vi "Emballage_BDD_choix_Config.vi"(8 "Error in":errorcluster caption="Error in (no error)") -> (0 "Error out":errorcluster, 1 "Arrêt programme?":bool=TRUE, 2 "Produit code FAS OUT":string, 3 "CLS_param_produit":T1)   [LabVIEW 2020]
uses:
  Emballage_BDD_param_Produit.ctl
  Choix_Config_ref.ctl
  Modules/FS/60_FS_Controles/60_FS_SetGet.ctl
  Labview emballage/enum_ON_OFF_Lecteur.ctl
  <vilib>/Utility/miscctls.llb/LVRowAndColumnUnsignedTypeDef.ctl
  <vilib>/drjdpowell/SQLite Library/SQL Connection/Open (path).vi
  <vilib>/drjdpowell/SQLite Library/SQL Connection/Open (string).vi
  <vilib>/AdvancedString/Path To Command Line String.vi
  <vilib>/drjdpowell/SQLite Library/SQL Connection/Connection.lvclass
panel:
  out "Indice Imprimante":i32
  in  "Port Com scan":u16(ring) items=["Autre", "FLATPROP"]
  out "imprimante Etiquettes":string(combo)="Sans_imprimante"
  out "Glissière":u8(slide) scale=0.0..100.0
  out "Dernière Synchro.":timestamp
  out "OK":bool
  in  "Bouton synchroniser":bool
  in  "Bouton Imprimante":bool
  in  "Bouton scanner":bool
  out "Produit code FAS":string
  out "sous-tableau":string[](array[string])
  in  "Bouton OK":bool
  in  "where valeur":string[](array[string])
  in  "Where colonne":string[](array[string])
  in  "stop":bool
  in  "Famille":u16(ring) items=["", "CHIPREG", "F011106", "F011107", "FASPROP", "FLATPROP", "NoTest", "S0020002", "S0020010", "S1121065", "S1121066", "S1121229", "S1121289", "S1121437", "S1210017", "S1220009", "S1220096"]
  in  "designation":u16(ring) items=["", "104mA_230Ohm", "138mA_130Ohm", "167mA 72ohm", "16mA_1152Ohm", "182mA_57Ohm", "186mA_14.4Ohm", "18V DC   4.50W", "18mA 288ohm", "211mA_57Ohm", "21mA 1152ohm", "21mA_1152Ohm", "23mA_576Ohm", "24V DC 4/0.40W", "258 SDGNUL  24V DC  14.50W", "264mA_36Ohm", "29mA 576ohm", "32mA 288ohm", "354mA_20Ohm", "36mA_230Ohm", "417mA_14.4Ohm", "4212 SDGNUL  24V DC  10W", "42mA 288ohm", "42mA_288Ohm", "48mA_130Ohm", "500mA_10Ohm", "59mA_288Ohm", "62mA_130Ohm", "83mA 72ohm", "83mA_72Ohm", "88mA_130Ohm", "BLOC  1P CHIPREG 10 l/min G1/8'' ", "BLOC  1P CHIPREG 10 l/min G1/8'' CLEAN ", "BLOC  1P CHIPREG 10 l/min M.MOUNT ", "BLOC  1P CHIPREG 10 l/min M.MOUNT CLEAN ", "BLOC  1P CHIPREG 500 ml/min G1/8 ", "BLOC  1P CHIPREG 500 ml/min G1/8 CLEAN ", "BLOC  1P CHIPREG 500 ml/min M.MOUNT ", "BLOC  1P CHIPREG 500 ml/min M.MOUNT CLEAN ", "BLOC  4P TAEMA EXTEND  24V / 5V DC", "BLOC 11-211P604-H0 4P 2 NIPPEL INJ ", "BLOC 2P TRILOGY ACTIVE EXHALATION CONTROL MODULE ", "BLOC 2X8P 3/2 NC NIPPEL ALU ", "BLOC 3P CALIBRATION UNIT ", "BLOC 4P EVU SN ELITE P4C HYBRID ", "BLOC 4P MANIFOLD VENTILATOR ", "BLOC 5P ARGON-N2 GASBOX FOR PQMS ", "BLOC 8P 3/2 NC NIPPEL ALU ", "BLOC DAGMAR DIGITAL ", "CARINA  AVEC FILTRE FERRITE ET GOUPILLE ", "CHIPREG MFC, 1 ls/min, RS232, G1/8, AIR, A-CLEAN ", "CHIPREG MFC, 1 ls/min, RS232, G1/8, AIR, STD MEDIC ", "CHIPREG MFC, 1 ls/min, RS232, M.MOUNT, AIR, A-CLEAN ", "CHIPREG MFC, 1 ls/min, RS232, M.MOUNT, AIR,STD MEDIC ", "CHIPREG MFC, 1 ls/min, RS485, G1/8, AIR, A-CLEAN ", "CHIPREG MFC, 1 ls/min, RS485, G1/8, AIR, STD MEDIC ", "CHIPREG MFC, 1 ls/min, RS485, M.MOUNT, AIR, A-CLEAN ", "CHIPREG MFC, 1 ls/min, RS485, M.MOUNT, AIR,STD MEDIC ", "CHIPREG MFC, 10 ls/min, RS232, G1/8, AIR, A-CLEAN ", "CHIPREG MFC, 10 ls/min, RS232, G1/8, AIR, STD MEDIC ", "CHIPREG MFC, 10 ls/min, RS232, M.MOUNT, AIR, A-CLEAN ", "CHIPREG MFC, 10 ls/min, RS232, M.MOUNT, AIR, STD MEDIC ", "CHIPREG MFC, 10 ls/min, RS485, G1/8, AIR, A-CLEAN ", "CHIPREG MFC, 10 ls/min, RS485, G1/8, AIR, STD MEDIC ", "CHIPREG MFC, 10 ls/min, RS485, M.MOUNT, AIR, A-CLEAN ", "CHIPREG MFC, 10 ls/min, RS485, M.MOUNT, AIR, STD MEDIC ", "CHIPREG MFC, 2 ls/min, RS232, G1/8, AIR, A-CLEAN ", "CHIPREG MFC, 2 ls/min, RS232, G1/8, AIR, STD MEDIC ", "CHIPREG MFC, 2 ls/min, RS232, M.MOUNT, AIR, A-CLEAN ", "CHIPREG MFC, 2 ls/min, RS232, M.MOUNT, AIR,STD MEDIC ", "CHIPREG MFC, 2 ls/min, RS485, G1/8, AIR, A-CLEAN ", "CHIPREG MFC, 2 ls/min, RS485, G1/8, AIR, STD MEDIC ", "CHIPREG MFC, 2 ls/min, RS485, M.MOUNT, AIR, A-CLEAN ", "CHIPREG MFC, 2 ls/min, RS485, M.MOUNT, AIR,STD MEDIC ", "CHIPREG MFC, 200 mls/min, RS232, G1/8, AIR, A-CLEAN ", "CHIPREG MFC, 200 mls/min, RS232, G1/8, AIR, STD MEDIC ", "CHIPREG MFC, 200 mls/min, RS232, M.MOUNT, AIR, A-CLEAN ", "CHIPREG MFC, 200 mls/min, RS232, M.MOUNT, AIR,STD MEDIC ", "CHIPREG MFC, 200 mls/min, RS485, G1/8, AIR, A-CLEAN ", "CHIPREG MFC, 200 mls/min, RS485, G1/8, AIR, STD MEDIC ", "CHIPREG MFC, 200 mls/min, RS485, M.MOUNT, AIR, A-CLEAN ", "CHIPREG MFC, 200 mls/min, RS485, M.MOUNT, AIR,STD MEDIC ", "CHIPREG MFC, 5 ls/min, RS232, G1/8, AIR, A-CLEAN ", "CHIPREG MFC, 5 ls/min, RS232, G1/8, AIR, STD MEDIC ", "CHIPREG MFC, 5 ls/min, RS232, M.MOUNT, AIR, A-CLEAN ", "CHIPREG MFC, 5 ls/min, RS232, M.MOUNT, AIR,STD MEDIC ", "CHIPREG MFC, 5 ls/min, RS485, G1/8, AIR, A-CLEAN ", "CHIPREG MFC, 5 ls/min, RS485, G1/8, AIR, STD MEDIC ", "CHIPREG MFC, 5 ls/min, RS485, M.MOUNT, AIR, A-CLEAN ", "CHIPREG MFC, 5 ls/min, RS485, M.MOUNT, AIR,STD MEDIC ", "CHIPREG MFC, 500 mls/min, RS232, G1/8, AIR, A-CLEAN ", "CHIPREG MFC, 500 mls/min, RS232, G1/8, AIR, STD MEDIC ", "CHIPREG MFC, 500 mls/min, RS232, M.MOUNT, AIR, A-CLEAN ", "CHIPREG MFC, 500 mls/min, RS232, M.MOUNT, AIR,STD MEDIC ", "CHIPREG MFC, 500 mls/min, RS485, G1/8, AIR, A-CLEAN ", "CHIPREG MFC, 500 mls/min, RS485, G1/8, AIR, STD MEDIC ", "CHIPREG MFC, 500 mls/min, RS485, M.MOUNT, AIR, A-CLEAN ", "CHIPREG MFC, 500 mls/min, RS485, M.MOUNT, AIR,STD MEDIC ", "DOSIERPATRONE (AUSTAUSCH-SET) ", "ENSEMBLE TORON EV PURGE & PEP ", "ENSEMBLE TORON EVS PEP N° KY724000 ", "ENSEMBLE TORON EVS PEP N° ST080387 D ", "Fluid control Current controller 211mA 24V IN4-20mA/IN10V ", "M06    18V DC   4.50W", "M06  5/1.5V DC 4.2/0.4W", "MODULE 1P CURRENT CTRL, SETPOINT 4-20mA ", "REVOLVER X6 "]
  in  "suffixe":u16(ring) items=["", "       ", "1110000", "1210000", "A      ", "D2MFIL", "D2WFIL", "D3MFIL", "D3MFIL ", "D3WD01 ", "D3WD05 ", "D3WD10 ", "D3WFIL", "D3WFIL ", "EQCFIL", "EQIFIL", "EQIMAX", "EQMLFT", "EQPFIL", "EQPLFT", "F011013", "F011014", "F011106", "F011107", "F011129", "F011363", "F01938 ", "F040340", "F040376", "F040427", "F04313 ", "F120014", "F120016", "F120017", "F120020", "F120023", "F120029", "F120030", "F120031", "F120039", "F120043", "F120044", "F120045", "F120047", "F120051", "F120058", "F120063", "F120064", "F120068", "F120072", "F120073", "F120074", "F120076", "F120077", "F120078", "F120083", "F120089", "F120090", "F120094", "F120096", "F120097", "F120098", "F120100", "F120101", "F120102", "F120103", "F120105", "F120106", "F120107", "F120108", "F120109", "F120110", "F120112", "F120113", "F120114", "F120115", "F120116", "F120118", "F120119", "F120120", "F120122", "F120123", "F120124", "F120126", "F120127", "F120128", "F120129", "F120130", "F120131", "F120132", "F120135", "F120136", "F120137", "F120138", "F120139", "F120140", "F120141", "F120142", "F120143", "F120144", "F120145", "F120146", "F120147", "F120148", "F120149", "F120150", "F120152", "F120153", "F120154", "F120155", "F120156", "F120157", "F120158", "F120159", "F120160", "F120161", "F120162", "F120163", "F120164", "F120165", "F120166", "F120167", "F120168", "F120169", "F120170", "F120171", "F120172", "F120174", "F120175", "F120176", "F120177", "F120178", "F120180", "F120181", "F120182", "F120183", "F120185", "F120187", "F120188", "F120190", "F120191", "F120192", "F120193", "F120194", "F120195", "F120196", "F120198", "F120199", "F120200", "F120201", "F120202", "F120203", "F120204", "F120206", "F120207", "F120212", "F120213", "F120214", "F120215", "F120216", "F120217", "F120218", "F120219", "F120220", "F120221", "F120222", "F120223", "F120224", "F120225", "F120226", "F120227", "F120228", "F120229", "F170001", "F170002", "F170003", "F170004", "F170005", "F170006", "F170007", "F170008", "F170009", "F170010", "F170011", "F170012", "F170013", "F170014", "F170015", "F170016", "F170017", "F170018", "F170019", "F170020", "F170021", "F170022", "IMIN30 ", "P170001", "P170002", "P170003", "f120205"]
  in  "No_Valve_FAS":u16(ring) items=["", "01-211-004-H1", "01-211E-01-H6", "01-211P-03-26", "01-213E-01-B6", "01-223E-01-B6", "04-331E-11-11", "04-341E-11-11", "12-216C-00-20", "12-216C-00-21", "12-216C-00-25", "12-216C-00-41", "12-216C-00-45", "12-216C-00-46", "12-216C-00120", "12-216C-00121", "12-216C-00141", "12-216C-00145", "12-216C-00146", "12-216C-00220", "12-216C-00221", "12-216C-00241", "12-216C-00245", "12-216C-00246", "12-216C-00321", "12-216C-00325", "12-216C-00341", "12-216C-01-20", "12-216C-01-21", "12-216C-01-25", "12-216C-01-41", "12-216C-01-45", "12-216C-01-46", "12-216C-01820", "12-216C-01821", "12-216C-02-20", "12-216C-02-21", "12-216C-02-25", "12-216C-02-41", "12-216C-02-45", "12-216C-02-46", "12-216C-03-20", "12-216C-03-21", "12-216C-03-25", "12-216C-03-41", "12-216C-03-45", "12-216C-04-20", "12-216C-04-21", "12-216C-04-25", "12-216C-04-40", "12-216C-04-41", "12-216C-04-45", "12-216C-04-46", "12-216C-04520", "12-216C-04521", "12-216C-04525", "12-216C-04540", "12-216C-04541", "12-216C-04545", "12-216C-04620", "12-216C-04621", "12-216C-04625", "12-216C-04640", "12-216C-04641", "12-216C-05141", "12-216E-01-25", "12-216P-00-20", "12-216P-00-21", "12-216P-00-41", "12-216P-00121", "12-216P-00220", "12-216P-00321", "12-216P-01-20", "12-216P-01-21", "12-216P-01821", "12-216P-02-20", "12-216P-02-21", "12-216P-02-45", "12-216P-03-20", "12-216P-03-21", "12-216P-04-20", "12-216P-04-21", "12-216P-04520", "12-216P-04521", "12-216P-04525", "12-216P-04541", "12-216V-04621", "17-211C-M0346", "17-211C-M0546", "17-216C-00-41", "17-216C-00-45", "17-216C-00-46", "17-216C-00141", "17-216C-00145", "17-216C-00146", "17-216C-00241", "17-216C-00245", "17-216C-00246", "17-216C-00341", "17-216C-00346", "17-216C-02-41", "17-216C-02-45", "17-216C-02-46", "17-216C-M0141", "17-216C-M0241", "17-216C-M0341", "17-216C-M0346", "17-216C-M0541", "17-216C-M0546", "17-216E100141", "17-216E100241", "17-216E100246", "17-216E200241", "17-216E200346", "17-216E300245", "40C2118CH----", "40M0011CG1811", "40M0011CG2811", "40M0011CJ1811", "40M0011CJ2811", "40M0021CG1811", "40M0021CG2811", "40M0021CJ1811", "40M0021CJ2811", "40M0051CG1811", "40M0051CG2811", "40M0051CJ1811", "40M0051CJ2811", "40M0101CG1811", "40M0101CG2811", "40M0101CJ1811", "40M0101CJ2811", "40M2002CG1811", "40M2002CG2811", "40M2002CJ1811", "40M2002CJ2811", "40M5002CG1811", "40M5002CG2811", "40M5002CJ1811", "40M5002CJ2811", "S002.0002", "S002.0008", "S002.0010", "S012.2051", "S112.1065", "S112.1066", "S112.1229", "S112.1289", "S112.1366", "S112.1437", "S112.1451", "S121.0017", "S122.0008", "S122.0009", "S122.0096", "S402.0001", "S402.0002", "S402.0003", "S402.0007", "S402.0008", "S402.0009", "S402.0010", "S402.0011", "S402.0012", "S402.0016"]
  in  "Liste multicolonne":i32(listbox)
  # "FILTRE:"
  # "SELECTIONNEZ LE PRODUIT:"
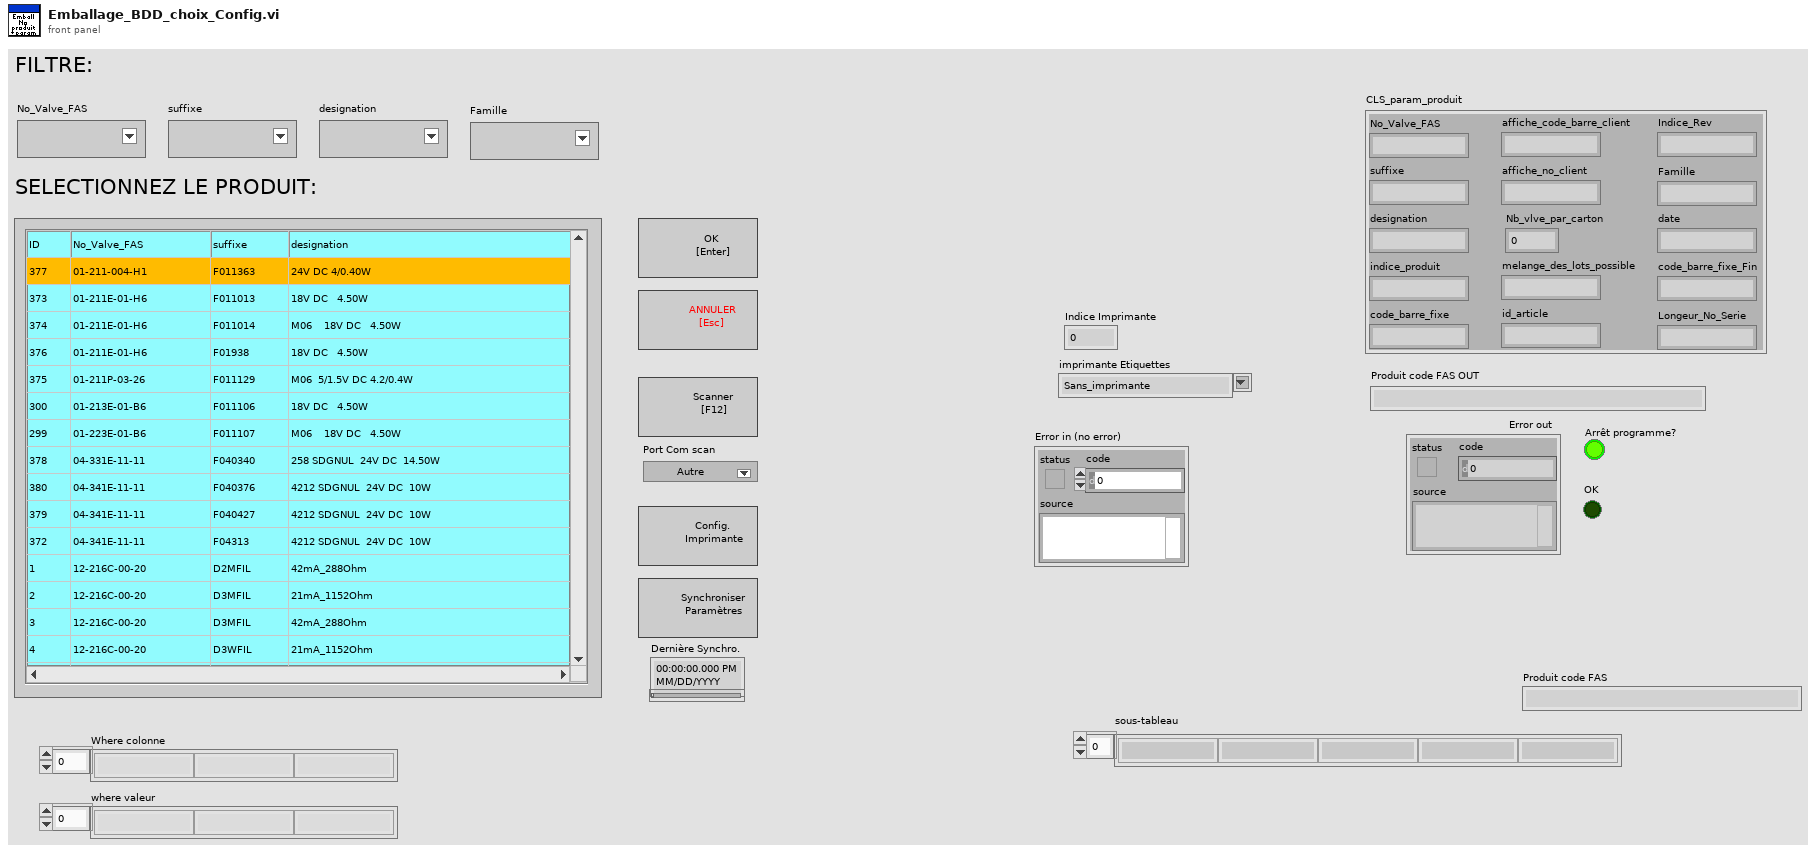
[diagram p1: front panel]
types:
  T1 = typedef "Emballage_BDD_param_Produit.ctl" = cluster{"No_Valve_FAS":string, "suffixe":string, "designation":string, "indice_produit":string, "code_barre_fixe":string, "affiche_code_barre_client":string, "affiche_no_client":string, "Nb_vlve_par_carton":u16, "melange_des_lots_possible":string, "id_article":string, "Indice_Rev":string, "Famille":string, "date":string, "code_barre_fixe_Fin":string, "Longeur_No_Serie":string}
  T2 = typedef "enum_ON_OFF_Lecteur.ctl" = enum16{"ON_COURT", "OFF", "ON", "OFF (open/Close)", "ON (open/close)"}
  T3 = typedef "LVRowAndColumnUnsignedTypeDef.ctl" = cluster{"Row":u32, "Column":u32}
  T4 = typedef "60_FS_SetGet.ctl" = enum16{"set", "get"}
  T5 = typedef "Choix_Config_ref.ctl" = cluster{"No_Valve_FAS":refnum<vi>, "Liste multicolonne":refnum<vi>, "suffixe":refnum<vi>, "designation":refnum<vi>, "Famille":refnum<vi>}
  T6 = typedef "60_FS_CLT_Chemins.ctl" = cluster{"Racine_local":path, "Racine_reseau":path, "Racine_Support_Application":path, "Fichier_Journalisation":path, "Connexion_BDD_VSX":path, "Connexion_BDD_PLZ":path}
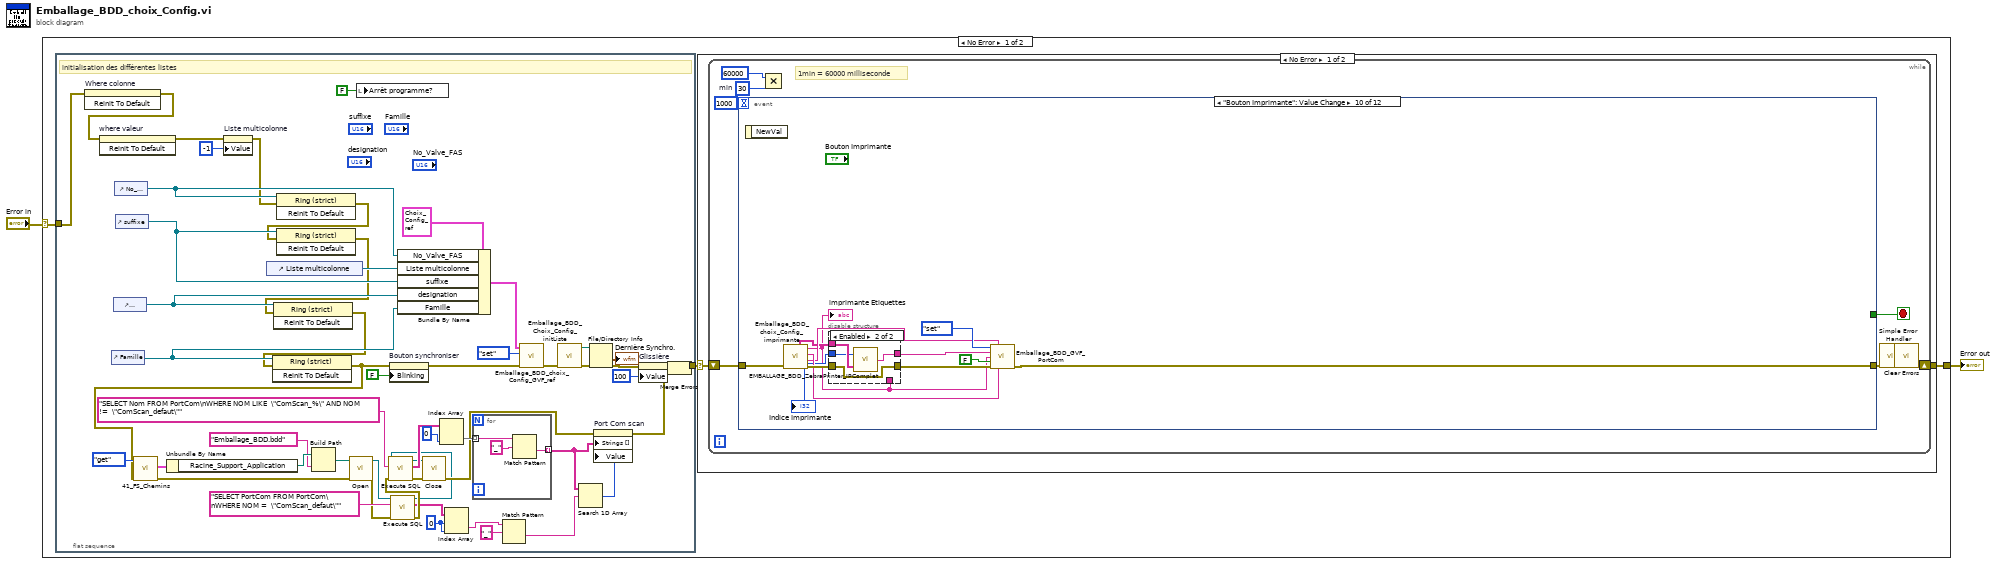
[diagram p0: block diagram]
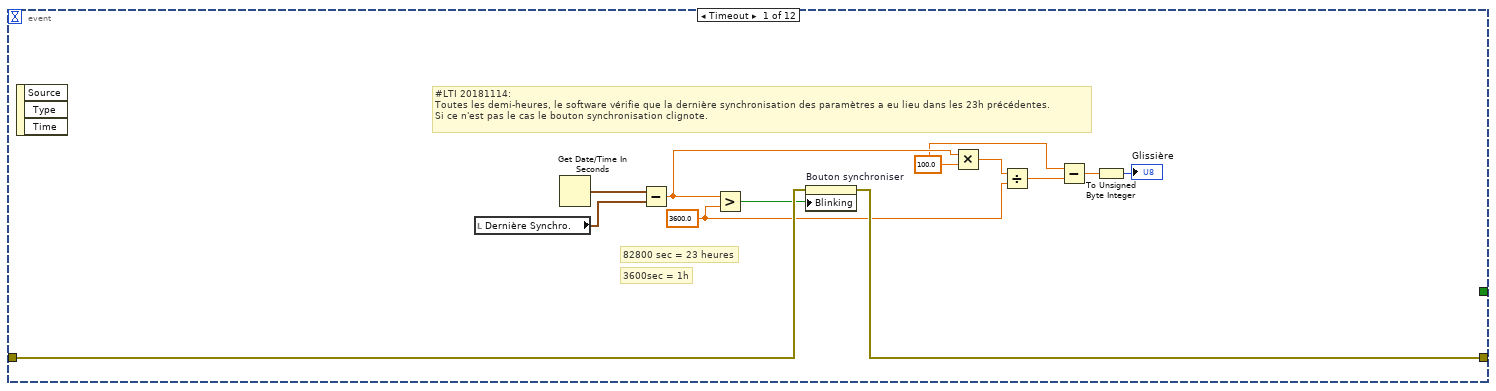
[diagram p2: hidden frame]
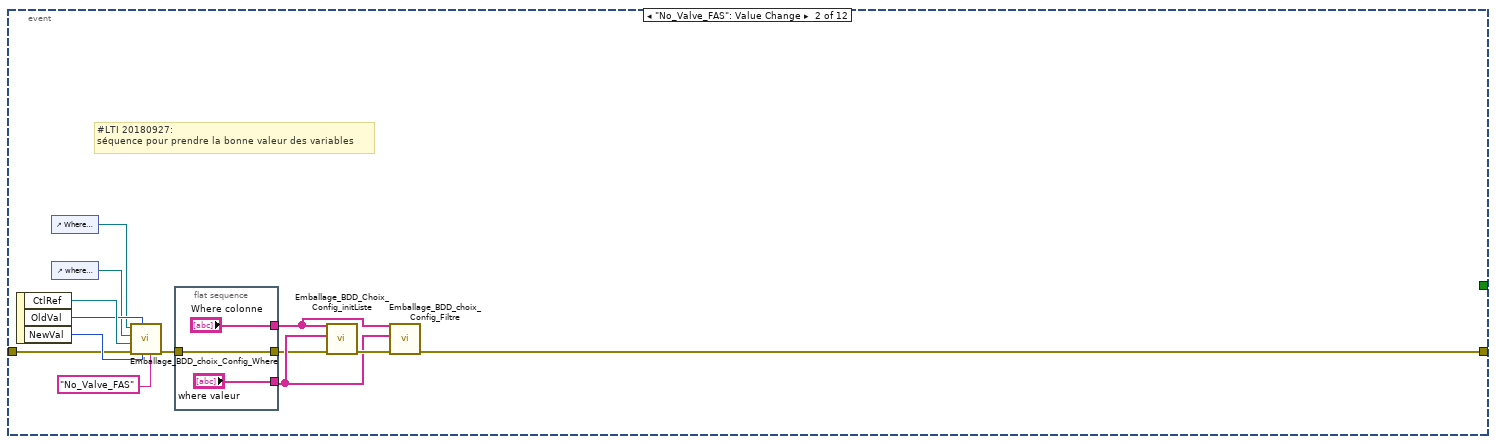
[diagram p3: hidden frame]
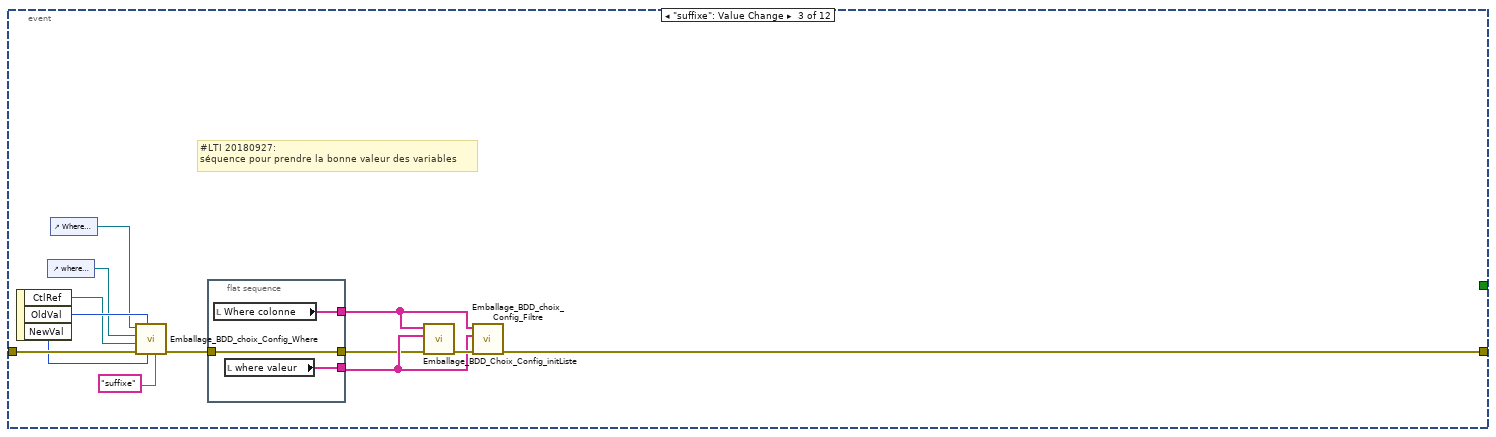
[diagram p4: hidden frame]
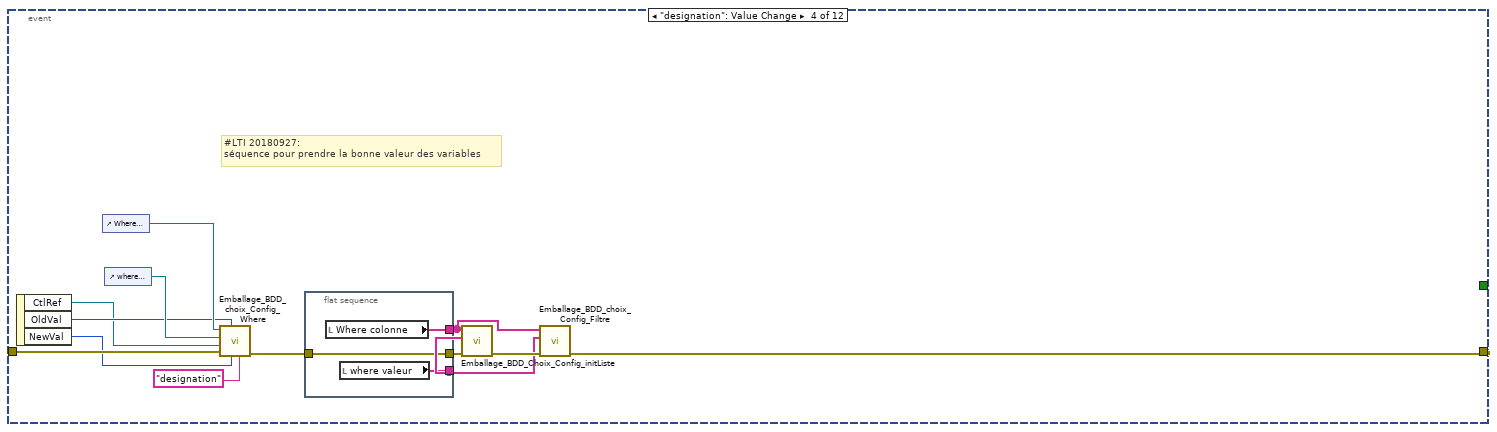
[diagram p5: hidden frame]
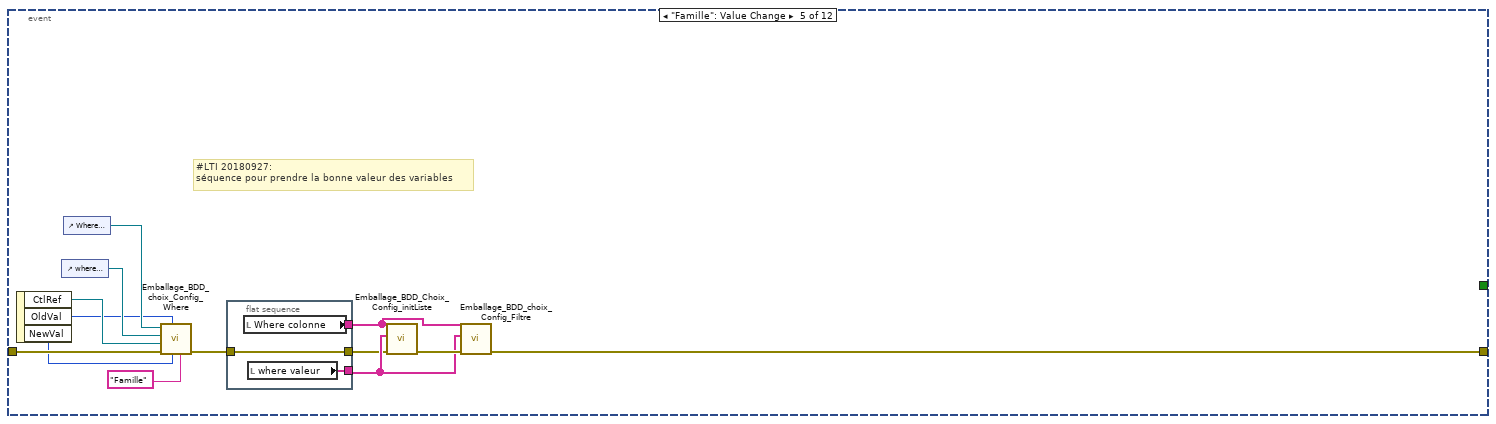
[diagram p6: hidden frame]
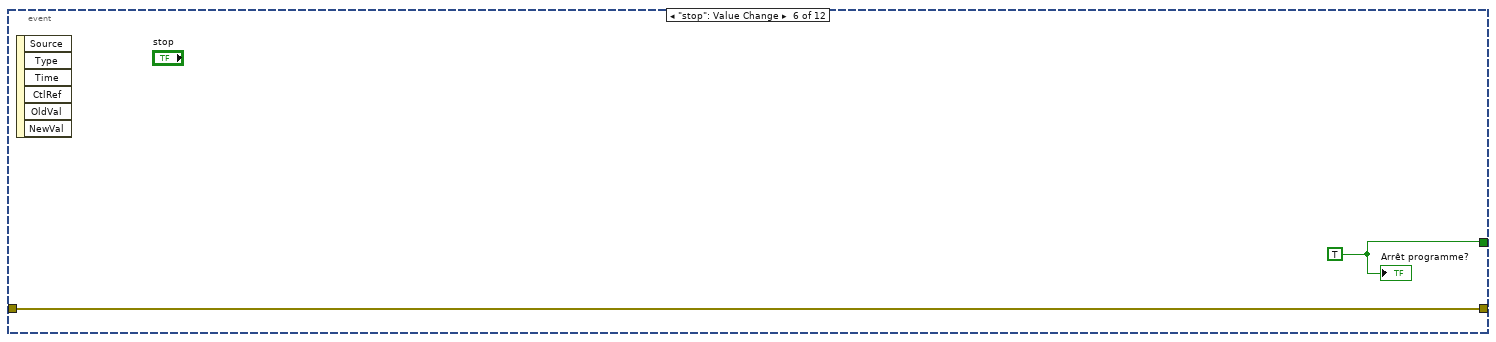
[diagram p7: hidden frame]
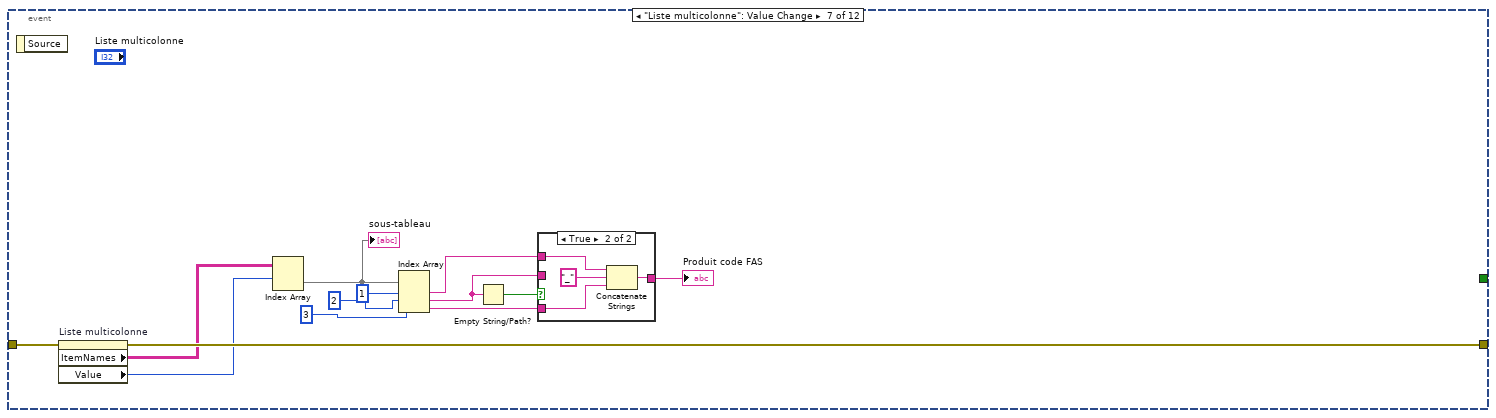
[diagram p8: hidden frame]
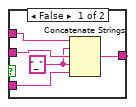
[diagram p9: hidden frame]
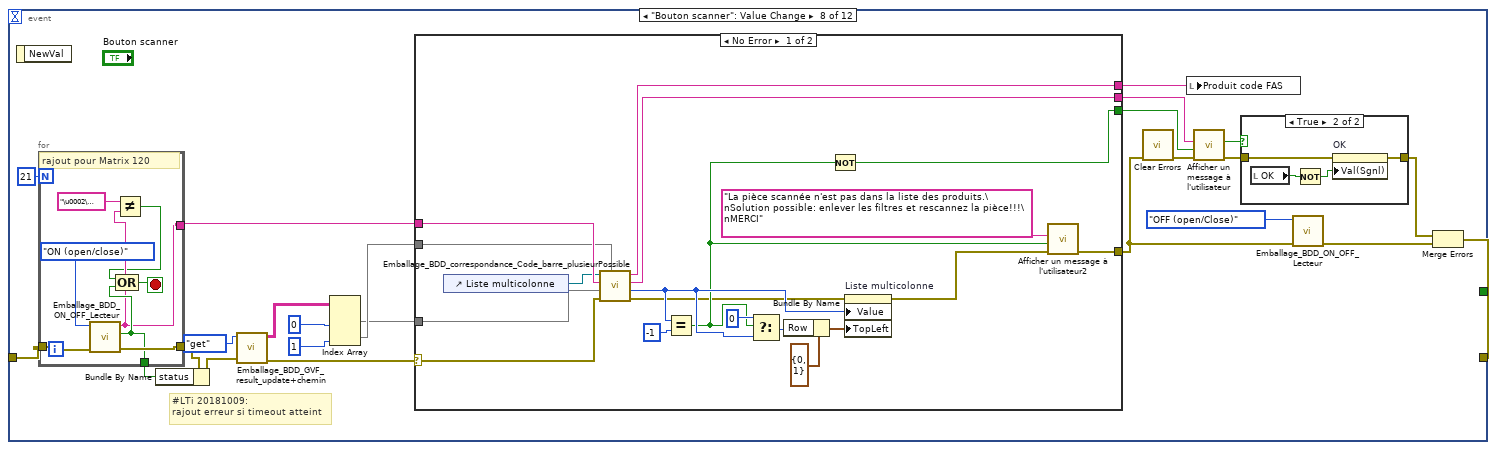
[diagram p10: hidden frame]
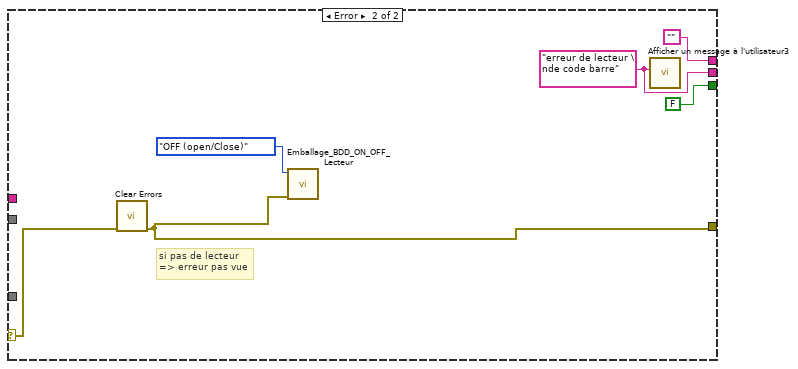
[diagram p12: hidden frame]
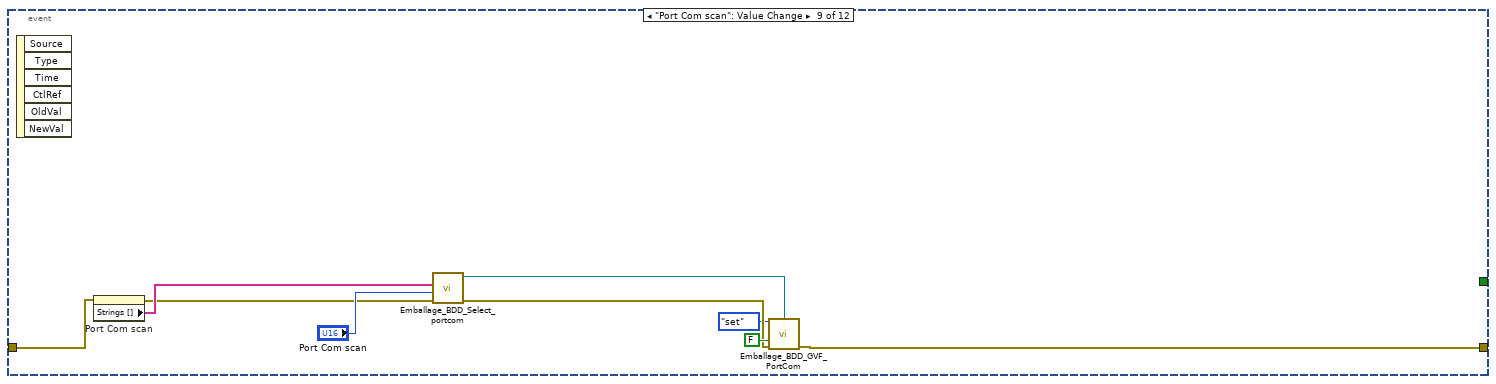
[diagram p13: hidden frame]
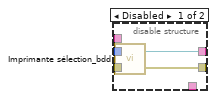
[diagram p14: hidden frame]
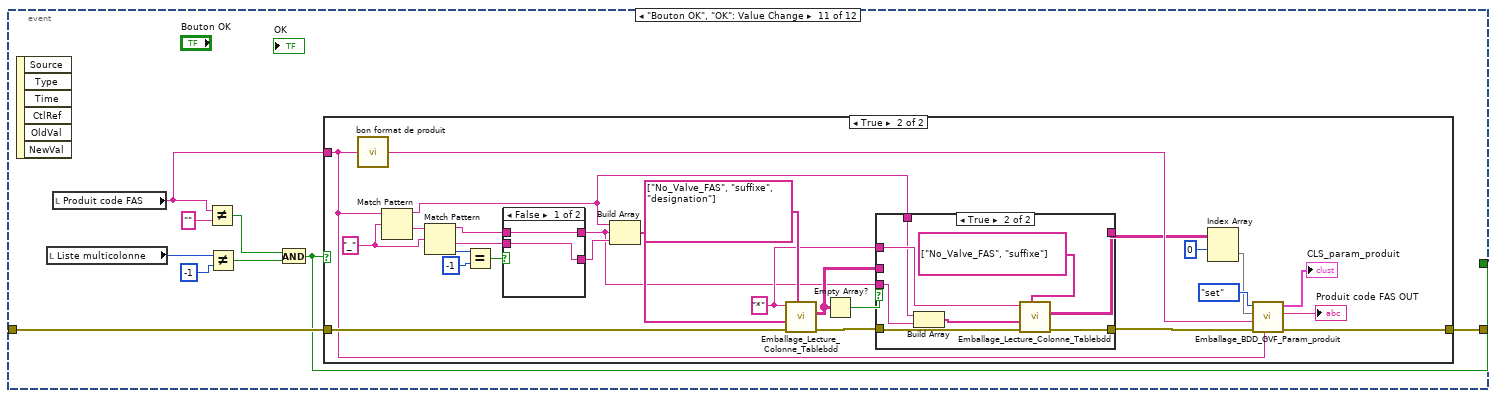
[diagram p15: hidden frame]
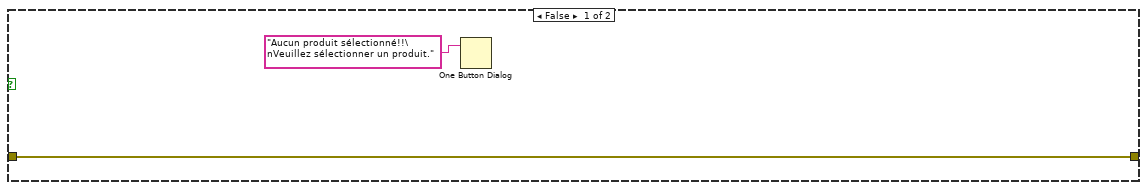
[diagram p16: hidden frame]
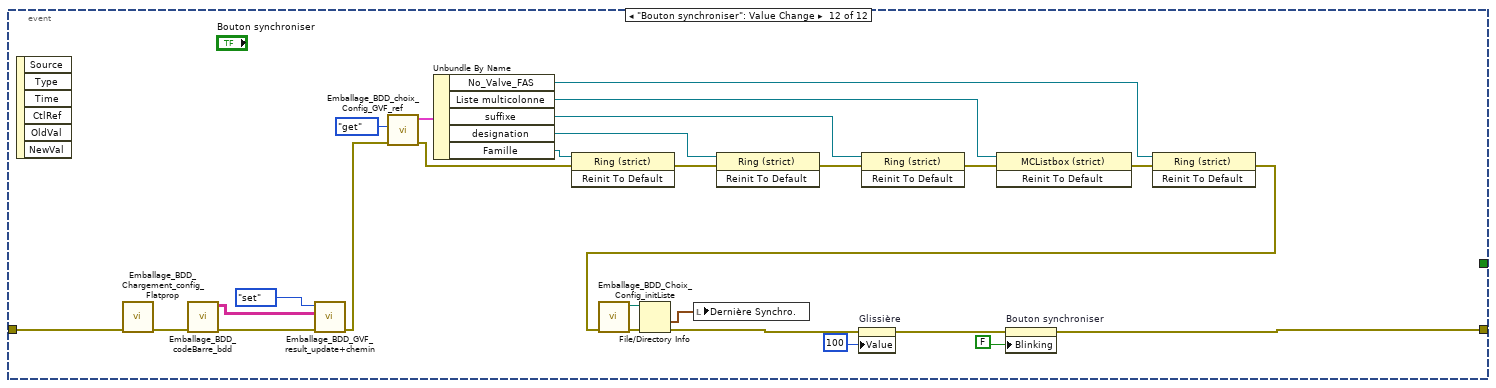
[diagram p19: hidden frame]
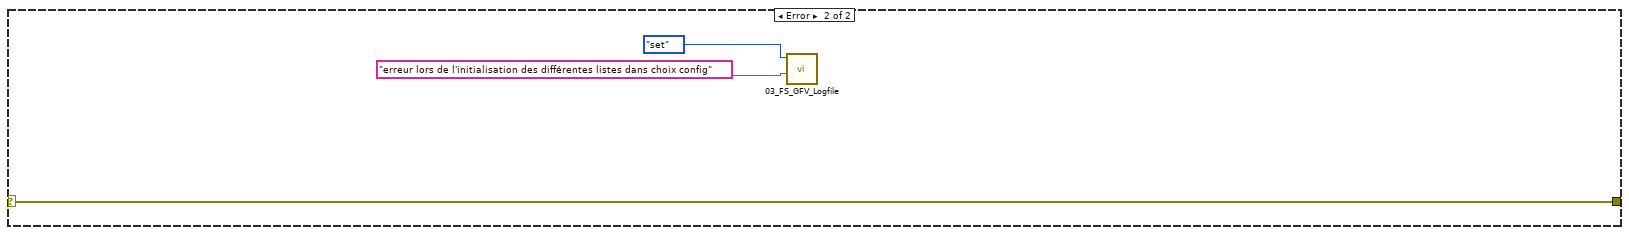
[diagram p20: hidden frame]
diagram:
  n1 = case shown="No Error" "Error in" {
    selector: "Error in" -> [w3 w345]
    tunnel: [w4 w345] -> w2
    frame No Error {
      n2 = flat-sequence {
        tunnel: w3 -> [w336]
        tunnel: [w301] -> w5
        frame #0 {
          w293 = 0 ("indice désactivé (col)")
          # "initialisation des différentes listes"
          n3 = invoke on="Where colonne" class="Tabl (strict)" method="Reinit To Default"(error in=w336) -> (error out=w331:errorcluster)  [unwired: 2 in, 2 out]
          n4 = invoke on="where valeur" class="Tabl (strict)" method="Reinit To Default"(error in=w331) -> (error out=w326:errorcluster)  [unwired: 2 in, 2 out]
          n5 = control-ref of="Famille"() -> (w332:refnum<vi>)
          n6 = control-ref of="designation"() -> (w333:refnum<vi>)
          n7 = control-ref of="No_Valve_FAS"() -> (w335:refnum<vi>)
          n8 = control-ref of="suffixe"() -> (w334:refnum<vi>)
          n9 = property on="Liste multicolonne" class="MCListbox (strict)"(error in=w326, "Value"=-1 ("Liste multicolonne")) -> (error out=w325:errorcluster)  [unwired: 1 in, 1 out]
          n10 = control-ref of="Liste multicolonne"() -> (w341:refnum<vi>)
          n11 = invoke class="Ring (strict)" method="Reinit To Default"(reference=w335, error in=w325) -> (error out=w330:errorcluster)  [unwired: 1 in, 2 out]
          n12 = invoke class="Ring (strict)" method="Reinit To Default"(reference=w334, error in=w330) -> (error out=w329:errorcluster)  [unwired: 1 in, 2 out]
          n13 = invoke class="Ring (strict)" method="Reinit To Default"(reference=w333, error in=w329) -> (error out=w328:errorcluster)  [unwired: 1 in, 2 out]
          n14 = invoke class="Ring (strict)" method="Reinit To Default"(reference=w332, error in=w328) -> (error out=w302:errorcluster)  [unwired: 1 in, 2 out]
          n15 = call "41_FS_Chemins.vi"("error in (no error)"=w302, "SetGet"=60_FS_SetGet."get") -> ("error out"=w310:errorcluster, "CLT_Chemins_out"=w308:T6)  [unwired: 8 in]
          n16 = Unbundle By Name(w308) -> ("Racine_Support_Application"=w309:path)
          n17 = Build Path(base path=w309, name or relative path="Emballage_BDD.bdd" ("nom ou chemin relatif")) -> (appended path=w311:path)
          n18 = call-poly <vilib>:"Open.vi"("error in (no error)"=w310, "db file"=w311) -> ("error out"=w296:errorcluster, "SQLite Connection"=w299:refnum<class "Connection.lvclass">)  [unwired: 8 in]
          n19 = local write "Arrêt programme?"(FALSE ("Arrêt programme")) -> ()
          n20 = property on="Bouton synchroniser" class="Bool"(error in=w302, "Blinking"=FALSE ("Clignotant")) -> (error out=w320:errorcluster)  [unwired: 1 in, 1 out]
          n21 = call <vilib>:"Execute SQL.vi"("error in (no error)"=w296, "SQL"="SELECT PortCom FROM PortCom\nWHERE NOM =  \"ComScan_defaut\"", "SQLite Connection in"=w299) -> ("error out"=w297:errorcluster, "Result Set"=w294:string[][], "SQLite Connection"=w295:refnum<class "Connection.lvclass">)  [unwired: 5 in, 1 out]
          n22 = call <vilib>:"Execute SQL.vi"("error in (no error)"=w297, "SQL"="SELECT Nom FROM PortCom\nWHERE NOM LIKE  \"ComScan_%\" AND NOM !=  \"ComScan_defaut\"", "SQLite Connection in"=w295) -> ("error out"=w313:errorcluster, "Result Set"=w314:string[][], "SQLite Connection"=w312:refnum<class "Connection.lvclass">)  [unwired: 5 in, 1 out]
          n23 = Bundle By Name(cluster=T5 {"No_Valve_FAS"=refnum, "Liste multicolonne"=refnum, "suffixe"=refnum, "designation"=refnum, "Famille"=refnum} ("Cluster IN"), "No_Valve_FAS"=w335, "Liste multicolonne"=w341, "suffixe"=w334, "designation"=w333, "Famille"=w332) -> (w340:T5)
          n24 = call-dynamic "Close.vi"("error in (no error)"=w313, "SQLite Connection in"=w312) -> ("error out"=w303:errorcluster)  [unwired: 9 in]
          n25 = Index Array(array=w314, index (col)=0 ("indice désactivé (col)")) -> (element=w315:string[])  [unwired: 1 in]
          n26 = Index Array(array=w294, index (row)=w293, index (col)=w293) -> (element=w291:string)
          n27 = for {
            tunnel: w315 -> [w343] mode=indexing
            tunnel: [w342] -> w290 mode=indexing
            n28 = Match Pattern(string=w343, regular expression="_" ("expression régulière")) -> (after substring=w342:string)  [unwired: 1 in, 3 out]
          }
          n29 = Match Pattern(string=w291, regular expression="_" ("expression régulière")) -> (after substring=w289:string)  [unwired: 1 in, 3 out]
          n30 = call "Emballage_BDD_choix_Config_GVF_ref.vi"("Error in"=w320, "Énum"=enum16{"get", "set"}."set", "Cluster IN"=w340) -> ("Error out"=w337:errorcluster)  [unwired: 7 in, 1 out]
          n31 = call "Emballage_BDD_Choix_Config_initListe.vi"("entrée d'erreur (pas d'erreur)"=w337) -> ("sortie d'erreur"=w323:errorcluster, "chemin complet"=w322:path)  [unwired: 9 in]
          n32 = Search 1D Array(1D array=w290, element=w289) -> (index of element=w288:i32)  [unwired: 1 in]
          n33 = File/Directory Info(path=w322, error in=w323) -> (last mod=→"Dernière Synchro.":timestamp, error out=w318:errorcluster)  [unwired: 5 out]
          n34 = property on="Port Com scan" class="Ring (strict)"(error in=w303, "Strings []"=w290, "Value"=w288) -> (error out=w300:errorcluster)  [unwired: 1 in, 1 out]
          n35 = property on="Glissière" class="Slide (strict)"(error in=w318, "Value"=u8 100 ("Glissière")) -> (error out=w317:errorcluster)  [unwired: 1 in, 1 out]
          n36 = Merge Errors(w317, w300) -> (w301:errorcluster)
        }
      }
      n37 = case shown="No Error" w5 {
        selector: w5 -> [w6 w287]
        tunnel: [w7 w287] -> w4
        frame No Error {
          n38 = while {
            shift-right: [w9] -> w7
            shift-left: w6 -> [w13]
            stop <- w15 stop-if-true
            w12 = 30  # min
            # "1min = 60000 milliseconde"
            n39 = event shown="[9] \"Bouton Imprimante\": Value Change" {
              selector: _ -> [_ _ _ _ _ _ _ _ _ _ _ _]
              dyn-events: _ -> [_ _ _ _ _ _ _ _ _ _ _ _]
              timeout: 1000 -> [_ _ _ _ _ _ _ _ _ _ _ _]
              tunnel: [_ _ _ _ _ w93 _ _ _ _ w209 _] -> w15
              tunnel: [w24 w32 w48 w64 w80 w92 w105 w120 w186 w196 w212 w279] -> w14
              tunnel: w13 -> [w25 w37 w55 w69 w85 w92 w106 w128 w184 w192 w213 w284]
              event Timeout {
                w16 = 100.0 ("y")
                w19 = 3600.0 ("y")
                # "3600sec = 1h"
                # "#LTI 20181114:\nToutes les demi-heures, le software vérifie que la dernière synchronisation des paramètres a eu lieu dans les 23h précédentes.\nSi ce n'est pas le cas le bouton synchronisation clignote."
                # "82800 sec = 23 heures"
                n40 = event-data() -> ()  [unwired: 1 in, 3 out]
                n41 = local read "Dernière Synchro."() -> (w26:timestamp)
                n42 = Get Date/Time In Seconds() -> (seconds since 1Jan1904=w27:timestamp)
                n43 = Subtract(x=w27, y=w26) -> (x-y=w22:dbl)
                n44 = Greater? ("Supérieur ?")(x=w22, y=w19) -> (0:w23:bool)
                n45 = property on="Bouton synchroniser" class="Bool"(error in=w25, "Blinking"=w23) -> (error out=w24:errorcluster)  [unwired: 1 in, 1 out]
                n46 = Multiply(x=w22, y=w16) -> (x*y=w21:dbl)
                n47 = Divide(x=w21, y=w19) -> (x/y=w18:dbl)
                n48 = Subtract(x=w16, y=w18) -> (x-y=w17:dbl)
                n49 = To Unsigned Byte Integer(number=w17) -> (unsigned 8bit integer=→"Glissière":u8)
              }
              event "No_Valve_FAS": Value Change {
                # "#LTI 20180927:\nséquence pour prendre la bonne valeur des variables"
                n50 = event-data() -> ("CtlRef"=w40:refnum<vi>, "OldVal"=w38:u16, "NewVal"=w39:u16)  [unwired: 1 in]
                n51 = control-ref of="Where colonne"() -> (w36:refnum<vi>)
                n52 = control-ref of="where valeur"() -> (w35:refnum<vi>)
                n53 = call "Emballage_BDD_choix_Config_Where.vi"("Nom_Colonne"="No_Valve_FAS", "NewVal"=w39, "OldVal"=w38, "entrée d'erreur (pas d'erreur)"=w37, "CtlRef"=w40, "referenceWhere valeur"=w35, "Array colonne"=w36) -> ("sortie d'erreur"=w28:errorcluster)  [unwired: 4 in]
                n54 = flat-sequence {
                  tunnel: ["Where colonne"] -> w31
                  tunnel: ["where valeur"] -> w30
                  tunnel: [w41] -> w29
                  tunnel: w28 -> [w41]
                  frame #0 {
                  }
                }
                n55 = call "Emballage_BDD_Choix_Config_initListe.vi"("entrée d'erreur (pas d'erreur)"=w29, "where valeur"=w30, "Where colonne"=w31) -> ("sortie d'erreur"=w33:errorcluster)  [unwired: 7 in, 1 out]
                n56 = call "Emballage_BDD_choix_Config_Filtre.vi"("Error in"=w33, "where valeur"=w30, "Where colonne"=w31) -> ("Error out"=w32:errorcluster)  [unwired: 8 in]
              }
              event "suffixe": Value Change {
                # "#LTI 20180927:\nséquence pour prendre la bonne valeur des variables"
                n57 = event-data() -> ("CtlRef"=w51:refnum<vi>, "OldVal"=w54:u16, "NewVal"=w50:u16)  [unwired: 1 in]
                n58 = control-ref of="where valeur"() -> (w52:refnum<vi>)
                n59 = control-ref of="Where colonne"() -> (w53:refnum<vi>)
                n60 = call "Emballage_BDD_choix_Config_Where.vi"("Nom_Colonne"="suffixe", "NewVal"=w50, "OldVal"=w54, "entrée d'erreur (pas d'erreur)"=w55, "CtlRef"=w51, "referenceWhere valeur"=w52, "Array colonne"=w53) -> ("sortie d'erreur"=w45:errorcluster)  [unwired: 4 in]
                n61 = flat-sequence {
                  tunnel: [w59] -> w47
                  tunnel: [w58] -> w46
                  tunnel: w45 -> [w57]
                  tunnel: [w57] -> w44
                  frame #0 {
                    n62 = local read "Where colonne"() -> (w59:string[])
                    n63 = local read "where valeur"() -> (w58:string[])
                  }
                }
                n64 = call "Emballage_BDD_Choix_Config_initListe.vi"("entrée d'erreur (pas d'erreur)"=w44, "where valeur"=w46, "Where colonne"=w47) -> ("sortie d'erreur"=w49:errorcluster)  [unwired: 7 in, 1 out]
                n65 = call "Emballage_BDD_choix_Config_Filtre.vi"("Error in"=w49, "where valeur"=w46, "Where colonne"=w47) -> ("Error out"=w48:errorcluster)  [unwired: 8 in]
              }
              event "designation": Value Change {
                # "#LTI 20180927:\nséquence pour prendre la bonne valeur des variables"
                n66 = event-data() -> ("CtlRef"=w66:refnum<vi>, "OldVal"=w68:u16, "NewVal"=w67:u16)  [unwired: 1 in]
                n67 = control-ref of="Where colonne"() -> (w71:refnum<vi>)
                n68 = control-ref of="where valeur"() -> (w72:refnum<vi>)
                n69 = call "Emballage_BDD_choix_Config_Where.vi"("Nom_Colonne"="designation", "NewVal"=w67, "OldVal"=w68, "entrée d'erreur (pas d'erreur)"=w69, "CtlRef"=w66, "referenceWhere valeur"=w72, "Array colonne"=w71) -> ("sortie d'erreur"=w60:errorcluster)  [unwired: 4 in]
                n70 = flat-sequence {
                  tunnel: [w75] -> w63
                  tunnel: [w74] -> w62
                  tunnel: [w73] -> w61
                  tunnel: w60 -> [w73]
                  frame #0 {
                    n71 = local read "Where colonne"() -> (w75:string[])
                    n72 = local read "where valeur"() -> (w74:string[])
                  }
                }
                n73 = call "Emballage_BDD_Choix_Config_initListe.vi"("entrée d'erreur (pas d'erreur)"=w61, "where valeur"=w62, "Where colonne"=w63) -> ("sortie d'erreur"=w65:errorcluster)  [unwired: 7 in, 1 out]
                n74 = call "Emballage_BDD_choix_Config_Filtre.vi"("Error in"=w65, "where valeur"=w62, "Where colonne"=w63) -> ("Error out"=w64:errorcluster)  [unwired: 8 in]
              }
              event "Famille": Value Change {
                # "#LTI 20180927:\nséquence pour prendre la bonne valeur des variables"
                n75 = event-data() -> ("CtlRef"=w84:refnum<vi>, "OldVal"=w83:u16, "NewVal"=w82:u16)  [unwired: 1 in]
                n76 = control-ref of="where valeur"() -> (w88:refnum<vi>)
                n77 = control-ref of="Where colonne"() -> (w87:refnum<vi>)
                n78 = call "Emballage_BDD_choix_Config_Where.vi"("Nom_Colonne"="Famille", "NewVal"=w82, "OldVal"=w83, "entrée d'erreur (pas d'erreur)"=w85, "CtlRef"=w84, "referenceWhere valeur"=w88, "Array colonne"=w87) -> ("sortie d'erreur"=w76:errorcluster)  [unwired: 4 in]
                n79 = flat-sequence {
                  tunnel: [w91] -> w79
                  tunnel: [w90] -> w78
                  tunnel: [w89] -> w77
                  tunnel: w76 -> [w89]
                  frame #0 {
                    n80 = local read "Where colonne"() -> (w91:string[])
                    n81 = local read "where valeur"() -> (w90:string[])
                  }
                }
                n82 = call "Emballage_BDD_Choix_Config_initListe.vi"("entrée d'erreur (pas d'erreur)"=w77, "where valeur"=w78, "Where colonne"=w79) -> ("sortie d'erreur"=w81:errorcluster)  [unwired: 7 in, 1 out]
                n83 = call "Emballage_BDD_choix_Config_Filtre.vi"("Error in"=w81, "where valeur"=w78, "Where colonne"=w79) -> ("Error out"=w80:errorcluster)  [unwired: 8 in]
              }
              event "stop": Value Change {
                w93 = TRUE
                n84 = event-data() -> ()  [unwired: 1 in, 6 out]
                "Arrêt programme?" <- w93
              }
              event "Liste multicolonne": Value Change {
                n85 = event-data() -> ()  [unwired: 1 in, 1 out]
                n86 = property on="Liste multicolonne" class="MCListbox (strict)"(error in=w106) -> (error out=w105:errorcluster, "ItemNames"=w104:string[][], "Value"=w96:i32)  [unwired: 1 in, 1 out]
                n87 = Index Array(array=w104, index (row)=w96) -> (element=w103:string[])  [unwired: 1 in]
                "sous-tableau" <- w103
                n88 = Index Array(array=w103, index #1=1 ("indice"), index #2=2 ("indice"), index #3=3 ("indice")) -> (element #1=w99:string, element #2=w94:string, element #3=w98:string)
                n89 = Empty String/Path?(string/path=w94) -> (empty?=w95:bool)
                n90 = case shown="True" w95 {
                  tunnel: w99 -> [w111 w112]
                  tunnel: w94 -> [w110 _]
                  tunnel: w98 -> [w109 w114]
                  tunnel: [w108 w115] -> w97
                  frame False {
                    w107 = "_"
                    n91 = Concatenate Strings(w111, w107, w110, w107, w109) -> (w108:string)
                  }
                  frame True {
                    n92 = Concatenate Strings(w112, "_", w114) -> (w115:string)
                  }
                }
                "Produit code FAS" <- w97
              }
              event "Bouton scanner": Value Change {
                # "#LTi 20181009:\nrajout erreur si timeout atteint"
                n93 = event-data() -> ()  [unwired: 1 in, 1 out]
                n94 = for {
                  N: 21 -> [_]
                  tunnel: [w141] -> w127
                  tunnel: [w143] -> w117
                  tunnel: w128 -> [w147]
                  tunnel: [w145] -> w126
                  stop <- w144 stop-if-true
                  # "rajout pour Matrix 120"
                  n95 = call "Emballage_BDD_ON_OFF_Lecteur.vi"("Error in"=w147, "ON/OFF lecteur"=enum_ON_OFF_Lecteur."ON (open/close)") -> ("Error out"=w145:errorcluster, "TIMEOUT_FIN?"=w143:bool, "Etiquette scanné"=w141:string)  [unwired: 7 in]
                  n96 = Not Equal?(x="\u0002\u0018", y=w141) -> (x != y?=w140:bool)
                  n97 = Compound Arithmetic op=OR ("Opérateur arithmétique")(w140, w143) -> (w144:bool)
                }
                n98 = Bundle By Name(cluster=w126, "status"=w117) -> (w118:errorcluster)
                n99 = call "Emballage_BDD_GVF_result_update+chemin.vi"("Error in"=w118, "Énum"=enum16{"get", "set"}."get") -> ("Error out"=w125:errorcluster, "Tab codif-code bar OUT"=w138:string[][])  [unwired: 8 in]
                n100 = Index Array(array=w138, index (col) #1=0 ("indice désactivé (col)"), index (col) #2=1 ("indice (col)")) -> (element #1=w134:string[], element #2=w135:string[])  [unwired: 2 in]
                n101 = case shown="No Error" w125 {
                  selector: w125 -> [w169 w174]
                  tunnel: [w155 w172] -> w123
                  tunnel: [w170 w175] -> w133
                  tunnel: w135 -> [w157 _]
                  tunnel: w127 -> [w158 _]
                  tunnel: w134 -> [w171 _]
                  tunnel: [w159 ""] -> w121
                  tunnel: [w160 FALSE] -> w131
                  frame No Error {
                    n102 = control-ref of="Liste multicolonne"() -> (w156:refnum<vi>)
                    n103 = call "Emballage_BDD_correspondance_Code_barre_plusieurPossible.vi"("tableau des codes barres"=w157, "entrée d'erreur\n (pas d'erreur)"=w169, "tableau des produits code FAS"=w171, "Etiquette scanné"=w158, "MulticolumnListbox en entrée"=w156) -> ("sortie d'erreur"=w154:errorcluster, "index_produit"=w163:i32, "message"=w170:string, "Produit Code FAS"=w159:string)  [unwired: 3 in]
                    n104 = Equal?(x=w163, y=-1) -> (x = y?=w161:bool)
                    n105 = Select(t=0 ("y"), s=w161, f=w163) -> (s? t:f=w167:i32)
                    n106 = Bundle By Name(cluster=T3 {"Row"=0, "Column"=1} ("Cellule visible en haut à gauche"), "Row"=w167) -> (w166:T3)
                    n107 = Not(x=w161) -> (.not. x?=w160:bool)
                    n108 = property on="Liste multicolonne" class="MCListbox (strict)"(error in=w154, "Value"=w163, "TopLeft"=w166) -> (error out=w153:errorcluster)  [unwired: 1 in, 1 out]
                    n109 = call "Afficher un message à l'utilisateur2"("error in (no error)"=w153, "Enable"=w161, "Message"="La pièce scannée n'est pas dans la liste des produits.\nSolution possible: enlever les filtres et rescannez la pièce!!!\nMERCI") -> ("error out"=w155:errorcluster)  [unwired: 7 in, 1 out]
                  }
                  frame Error {
                    w175 = "erreur de lecteur \nde code barre"
                    # "si pas de lecteur\n=> erreur pas vue"
                    n110 = call <vilib>:"Clear Errors.vi"("error in (no error)"=w174) -> ("error out"=w172:errorcluster)  [unwired: 5 in, 1 out]
                    n111 = call "Emballage_BDD_ON_OFF_Lecteur.vi"("Error in"=w172, "ON/OFF lecteur"=enum_ON_OFF_Lecteur."OFF (open/Close)") -> ()  [unwired: 7 in, 3 out]
                    n112 = call "Afficher un message à l'utilisateur3"("Message"=w175) -> ()  [unwired: 9 in, 2 out]
                  }
                }
                n113 = call <vilib>:"Clear Errors.vi"("error in (no error)"=w123) -> ("error out"=w132:errorcluster)  [unwired: 5 in, 1 out]
                n114 = local write "Produit code FAS"(w121) -> ()
                n115 = call "Afficher un message à l'utilisateur"("error in (no error)"=w132, "Enable"=w131, "Message"=w133) -> ("error out"=w129:errorcluster, "OUI"=w130:bool)  [unwired: 7 in]
                n116 = case shown="True" w130 {
                  tunnel: w129 -> [w148 w152]
                  tunnel: [w148 w149] -> w119
                  frame False {
                  }
                  frame True {
                    n117 = local read "OK"() -> (w151:bool)
                    n118 = Not(x=w151) -> (.not. x?=w150:bool)
                    n119 = property on="OK" class="Bool (strict)"(error in=w152, "Val(Sgnl)"=w150) -> (error out=w149:errorcluster)  [unwired: 1 in, 1 out]
                  }
                }
                n120 = call "Emballage_BDD_ON_OFF_Lecteur.vi"("Error in"=w123, "ON/OFF lecteur"=enum_ON_OFF_Lecteur."OFF (open/Close)") -> ("Error out"=w122:errorcluster)  [unwired: 7 in, 2 out]
                n121 = Merge Errors(w119, w122) -> (w120:errorcluster)
              }
              event "Port Com scan": Value Change {
                n122 = event-data() -> ()  [unwired: 1 in, 6 out]
                n123 = property on="Port Com scan" class="Ring (strict)"(error in=w184) -> (error out=w179:errorcluster, "Strings []"=w183:string[])  [unwired: 1 in, 1 out]
                n124 = call "Emballage_BDD_Select_portcom.vi"("entrée d'erreur (pas d'erreur)"=w179, "Famille"="Port Com scan", "Familles"=w183) -> ("sortie d'erreur"=w180:errorcluster, "Refnum VISA en sortie"=w181:refnum<visa-resource-name>)  [unwired: 7 in]
                n125 = call "Emballage_BDD_GVF_PortCom.vi"("Énum"=enum16{"get", "set"}."set", "PortCom Scanner IN"=w181, "bdd"=FALSE, "Error in"=w180) -> ("Error out"=w186:errorcluster)  [unwired: 5 in, 6 out]
              }
              event "Bouton Imprimante": Value Change {
                n126 = event-data() -> ()  [unwired: 1 in, 1 out]
                n127 = call "Emballage_BDD_choix_Config_imprimante.vi"("Error in"=w192) -> ("Error out"=w198:errorcluster, "imprimante Certificats 2"=w190:string, "Dec. Droite"=w191:string, "imprimante Etiquettes OUT"=w187:string, "Indice Imprimante"=w188:i32, "Liste IP"=w189:string[])  [unwired: 5 in]
                "imprimante Etiquettes" <- w187
                "Indice Imprimante" <- w188
                n128 = disable-structure shown="Enabled" {
                  disable-tunnel: w198 -> [w201 w205]
                  disable-tunnel: [w200 w205] -> w197
                  disable-tunnel: [w199 w204] -> w194
                  disable-tunnel: w189 -> [_ w203]
                  disable-tunnel: w188 -> [_ w202]
                  disable-tunnel: w187 -> [_ _]
                  frame Disabled {
                    n129 = call "Imprimante sélection_bdd.vi"("entrée d'erreur"=w201) -> ("sortie d'erreur"=w200:errorcluster, "Output ressource VISA"=w199:refnum<visa-resource-name>)  [unwired: 1 in]
                  }
                  frame Enabled {
                    n130 = call "EMBALLAGE_BDD_ZebraPrinter_IPComplet.vi"("Liste IP"=w203, "indice"=w202) -> ("IP Zebra complet"=w204:string)
                  }
                }
                n131 = call "Emballage_BDD_GVF_PortCom.vi"("Énum"=enum16{"get", "set"}."set", "Imprimante certif. IN"=w190, "PortCom imprimante IN"=w194, "Imprimante Zebra IN"=w187, "bdd"=FALSE, "Error in"=w197, "DecDroit_IN"=w191) -> ("Error out"=w196:errorcluster)  [unwired: 2 in, 6 out]
              }
              event "Bouton OK", "OK": Value Change {
                n132 = event-data() -> ()  [unwired: 1 in, 6 out]
                n133 = local read "Liste multicolonne"() -> (w208:i32)
                n134 = local read "Produit code FAS"() -> (w210:string)
                n135 = Not Equal?(x=w210, y="") -> (x != y?=w211:bool)
                n136 = Not Equal?(x=w208, y=-1) -> (x != y?=w206:bool)
                n137 = And(x=w211, y=w206) -> (x .and. y?=w209:bool)
                n138 = case shown="True" w209 {
                  tunnel: w213 -> [w216 w240]
                  tunnel: [w216 w237] -> w212
                  tunnel: w210 -> [_ w217]
                  frame False {
                    n139 = One Button Dialog(message="Aucun produit sélectionné!!\nVeuillez sélectionner un produit.") -> ()  [unwired: 1 in, 1 out]
                  }
                  frame True {
                    w220 = "*" ("Colonne")
                    w241 = "_" ("expression régulière")
                    n140 = call "bon format de produit.vi"("Chaîne"=w217) -> ("Chaîne 2"=w234:string)
                    n141 = Match Pattern(string=w217, regular expression=w241) -> (before substring=w219:string, after substring=w242:string)  [unwired: 1 in, 2 out]
                    n142 = Match Pattern(string=w242, regular expression=w241) -> (before substring=w230:string, after substring=w229:string, offset past match=w233:i32)  [unwired: 1 in, 1 out]
                    n143 = Equal?(x=w233, y=-1) -> (x = y?=w231:bool)
                    n144 = case shown="False" w231 {
                      tunnel: [w255 w256] -> w218
                      tunnel: w230 -> [w255 w257]
                      tunnel: w229 -> [w254 w256]
                      tunnel: [w254 w257] -> w228
                      frame False {
                      }
                      frame True {
                      }
                    }
                    n145 = Build Array(w219, w218, w228) -> (w226:string[])
                    n146 = call "Emballage_Lecture_Colonne_Tablebdd.vi"("Where colonne"=string[] ["No_Valve_FAS", "suffixe", "designation"], "Error in"=w240, "where valeur"=w226, "Colonne"=w220) -> ("Error out"=w225:errorcluster, "Result Set"=w222:string[][])  [unwired: 4 in, 2 out]
                    n147 = Empty Array?(array=w222) -> (empty?=w223:bool)
                    n148 = case shown="True" w223 {
                      tunnel: w225 -> [w244 w253]
                      tunnel: [w244 w252] -> w224
                      tunnel: [w245 w250] -> w221
                      tunnel: w222 -> [w245 _]
                      tunnel: w220 -> [_ w251]
                      tunnel: w219 -> [_ w248]
                      tunnel: w218 -> [_ w247]
                      frame False {
                      }
                      frame True {
                        n149 = Build Array(w248, w247) -> (w249:string[])
                        n150 = call "Emballage_Lecture_Colonne_Tablebdd.vi"("Where colonne"=string[] ["No_Valve_FAS", "suffixe"], "Error in"=w253, "where valeur"=w249, "Colonne"=w251) -> ("Error out"=w252:errorcluster, "Result Set"=w250:string[][])  [unwired: 4 in, 2 out]
                      }
                    }
                    n151 = Index Array(array=w221, index (row)=0 ("indice (ligne)")) -> (element=w227:string[])  [unwired: 1 in]
                    n152 = call "Emballage_BDD_GVF_Param_produit.vi"("Produit_Formate IN"=w217, "Error in"=w224, "Produit IN"=w234, "Tableau param produit"=w227, "Énum"=enum16{"set", "get"}."set") -> ("Error out"=w237:errorcluster, "Produit OUT"=→"Produit code FAS OUT":string, "CLS_param_produit"=→"CLS_param_produit":T1)  [unwired: 3 in, 1 out]
                  }
                }
              }
              event "Bouton synchroniser": Value Change {
                n153 = event-data() -> ()  [unwired: 1 in, 6 out]
                n154 = call "Emballage_BDD_Chargement_config_Flatprop.vi"("Error in"=w284) -> ("Error out"=w283:errorcluster)  [unwired: 10 in]
                n155 = call "Emballage_BDD_codeBarre_bdd.vi"("Error in"=w283) -> ("Error out"=w282:errorcluster, "tableau ajouté"=w280:string[][])  [unwired: 9 in]
                n156 = call "Emballage_BDD_GVF_result_update+chemin.vi"("Error in"=w282, "Tab codif-code bar IN"=w280, "Énum"=enum16{"get", "set"}."set") -> ("Error out"=w269:errorcluster)  [unwired: 7 in, 1 out]
                n157 = call "Emballage_BDD_choix_Config_GVF_ref.vi"("Error in"=w269, "Énum"=enum16{"get", "set"}."get") -> ("Error out"=w266:errorcluster, "Cluster OUT"=w273:T5)  [unwired: 8 in]
                n158 = Unbundle By Name(w273) -> ("No_Valve_FAS"=w270:refnum<vi>, "Liste multicolonne"=w267:refnum<vi>, "suffixe"=w271:refnum<vi>, "designation"=w272:refnum<vi>, "Famille"=w274:refnum<vi>)
                n159 = invoke class="Ring (strict)" method="Reinit To Default"(reference=w274, error in=w266) -> (error out=w265:errorcluster)  [unwired: 1 in, 2 out]
                n160 = invoke class="Ring (strict)" method="Reinit To Default"(reference=w272, error in=w265) -> (error out=w264:errorcluster)  [unwired: 1 in, 2 out]
                n161 = invoke class="Ring (strict)" method="Reinit To Default"(reference=w271, error in=w264) -> (error out=w263:errorcluster)  [unwired: 1 in, 2 out]
                n162 = invoke class="MCListbox (strict)" method="Reinit To Default"(reference=w267, error in=w263) -> (error out=w262:errorcluster)  [unwired: 1 in, 2 out]
                n163 = invoke class="Ring (strict)" method="Reinit To Default"(reference=w270, error in=w262) -> (error out=w261:errorcluster)  [unwired: 1 in, 2 out]
                n164 = call "Emballage_BDD_Choix_Config_initListe.vi"("entrée d'erreur (pas d'erreur)"=w261) -> ("sortie d'erreur"=w276:errorcluster, "chemin complet"=w277:path)  [unwired: 9 in]
                n165 = File/Directory Info(path=w277, error in=w276) -> (last mod=w275:timestamp, error out=w259:errorcluster)  [unwired: 5 out]
                n166 = local write "Dernière Synchro."(w275) -> ()
                n167 = property on="Glissière" class="Slide (strict)"(error in=w259, "Value"=u8 100 ("Glissière")) -> (error out=w258:errorcluster)  [unwired: 1 in, 1 out]
                n168 = property on="Bouton synchroniser" class="Bool"(error in=w258, "Blinking"=FALSE ("Clignotant")) -> (error out=w279:errorcluster)  [unwired: 1 in, 1 out]
              }
            }
            n169 = Multiply(x=60000, y=w12) -> ()  [unwired: 1 out]
            n170 = call <vilib>:"Simple Error Handler.vi"("error in (no error)"=w14) -> ("error out"=w8:errorcluster)  [unwired: 4 in, 4 out]
            n171 = call <vilib>:"Clear Errors.vi"("error in (no error)"=w8) -> ("error out"=w9:errorcluster)  [unwired: 5 in, 1 out]
          }
        }
        frame Error {
          n172 = call "03_FS_GFV_Logfile.vi"("Chaîne"="erreur lors de l'initialisation des différentes listes dans choix config", "States"=60_FS_SetGet."set") -> ()  [unwired: 8 in, 2 out]
        }
      }
    }
    frame Error {
      n173 = call "03_FS_GFV_Logfile.vi"("Chaîne"="Erreur avant Choix_Config", "States"=60_FS_SetGet."set") -> ()  [unwired: 8 in, 2 out]
    }
  }
  "Error out" <- w2
